vi "Disarm.vi"(8 "error in (no error)":errorcluster, 9 "Request type":T1, 10 "Requester":string, 11 "Pulse Recorder in":refnum<class "Pulse Recorder.lvclass">) -> (0 "error out":errorcluster, 3 "Pulse Recorder out":refnum<class "Pulse Recorder.lvclass">)   [LabVIEW 2021, in "Pulse Recorder.lvclass"]
uses:
  Pulse Recorder.lvclass
  Controllers/Process Controller/Request type.ctl
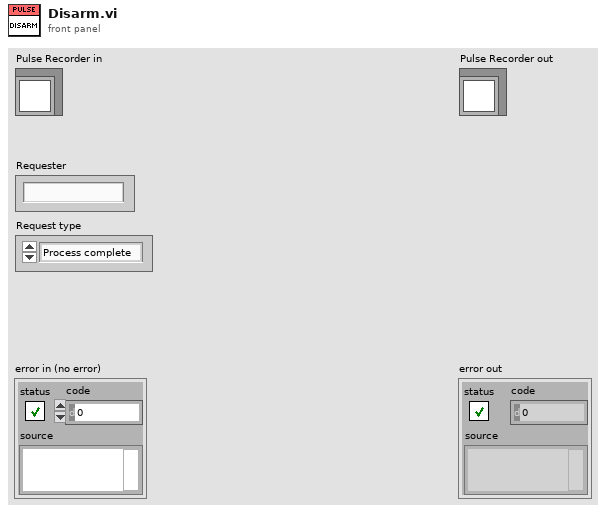
[diagram p1: front panel]
types:
  T1 = typedef "Request type.ctl" = enum16{"Process complete", "User command", "Auto-restart", "Error"}
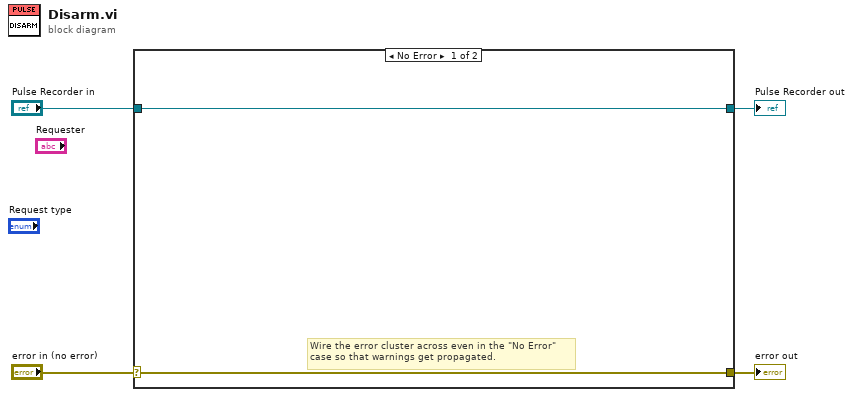
[diagram p0: block diagram]
diagram:
  n1 = case shown="No Error" "error in (no error)" {
    selector: "error in (no error)" -> [w5 w8]
    tunnel: [w5 w8] -> w3
    tunnel: [w6 w7] -> w1
    tunnel: "Pulse Recorder in" -> [w6 w7]
    frame No Error {
      # "Wire the error cluster across even in the \"No Error\"\ncase so that warnings get propagated."
    }
    frame Error {
    }
  }
  "error out" <- w3
  "Pulse Recorder out" <- w1
